vi "readLUT.vi"(8 "error in (no error)":errorcluster, 11 "AOTF in":refnum<class "AOTF.lvclass">) -> (0 "error out":errorcluster, 3 "AOTF out":refnum<class "AOTF.lvclass">)   [LabVIEW 2012, in "AOTF.lvclass"]
uses:
  AOTF.lvclass
  AOTF.lvclass/AOTF.ctl
  <vilib>/Utility/file.llb/Read From Spreadsheet File (DBL).vi
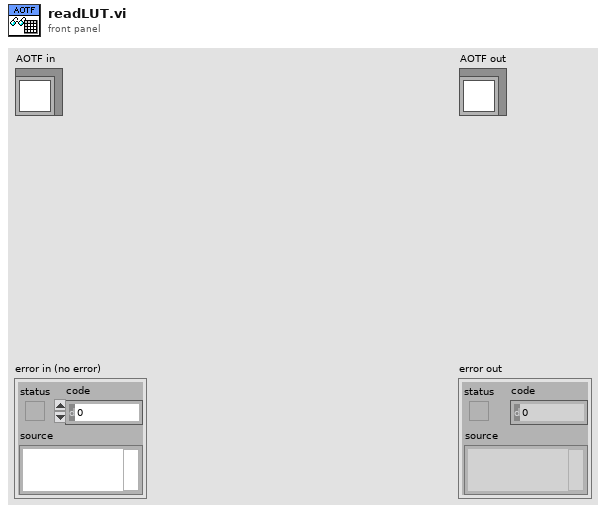
[diagram p1: front panel]
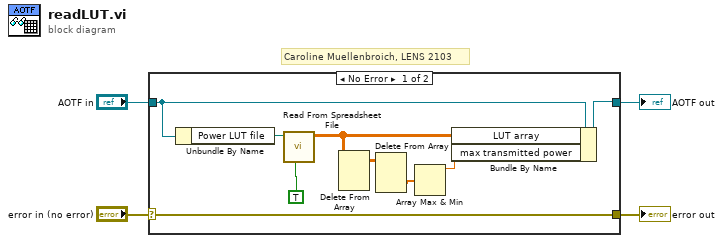
[diagram p0: block diagram]
diagram:
  # "Caroline Muellenbroich, LENS 2103"
  n1 = case shown="No Error" "error in (no error)" {
    selector: "error in (no error)" -> [w13 w15]
    tunnel: [w13 w15] -> w3
    tunnel: [w9 w14] -> w1
    tunnel: "AOTF in" -> [w10 w14]
    frame No Error {
      n2 = Unbundle By Name(w10) -> ("Power LUT file"=w11:path)
      n3 = call-poly <vilib>:"Read From Spreadsheet File.vi"("transpose (no:F)"=TRUE, "file path (dialog if empty)"=w11) -> ("all rows"=w8:dbl[][])  [unwired: 5 in, 4 out]
      n4 = Delete From Array(array=w8) -> (array with subset deleted=w7:dbl[][])  [unwired: 3 in, 1 out]
      n5 = Delete From Array(array=w7) -> (deleted portion=w6:dbl[])  [unwired: 3 in, 1 out]
      n6 = Array Max & Min(array=w6) -> (max value=w5:dbl)  [unwired: 3 out]
      n7 = Bundle By Name(cluster=w10, "LUT array"=w8, "max transmitted power"=w5) -> (w9:refnum<class "AOTF.lvclass">)
    }
    frame Error {
    }
  }
  "error out" <- w3
  "AOTF out" <- w1
